vi "Main_MaintenanceCounters_EventDriven.vi"() -> ()   [LabVIEW 2017]
uses:
  <vilib>/Utility/file.llb/Write Delimited Spreadsheet (string).vi
panel:
  in  "SignaiFromPLC":bool[](array[boolean])
  out "CycleTimeCluster":T1
  out "Table Control":string[][](table)
  out "ConnectionCluster":cluster{"Connection":bool, "MachineName":string}
  out "UDT_1":T2
  in  "CountersConfiguration":T3
  out "CountersConfigMerged":T4(array[cluster])
  out "CounterLineName Path":path
  in  "stop":bool
  in  "Tab":T5(tab)
  in  "Sort":bool
  in  "ResetAlarm":bool[](array[boolean])
  out "ArrayAlarm":bool[](array[boolean])
  out "OnlineStations":T6(array[cluster])
  in  "Counters Monitor Array":T7(array[cluster])
  in  "RefreshCurrentCounter":bool
  in  "SaveCurrentCounter":bool
  out "CurrentCountersPath":path
  in  "Count Signal":bool[](array[boolean])
  out "CycleTimeMonitor":T8(array[cluster])
  out "CycleTimePath":path
  in  "CountersConfigArray":T4(array[cluster]) {"StoppageAlarmCounter" format="%#_6f"; "PreparationAlarmCounter" format="%#_6f"}
  in  "RefreshCountersConfig":bool
  in  "SaveCountersConfig":bool
  out "Counters Configuration Path":path
  in  "MachineNameID":u16(ring) items=["MA520", "MA500", "MA490", "MA475", "MA470"]
  out "Red":dbl
  out "Yellow":dbl
  out "Green":dbl
  out "Line Name":string
  in  "PLC Connection Array":T9(array[cluster]) {"MemoryType" items=["CR (Control Relay)", "MR (Internal Auxiliary Relay)", "VB (Work Relay)", "LR (Latch Relay)", "B (Link Relay)", "R (Relay)", "DM (Data Memory)", "EM (Extended Data Memory)", "FM (File Register 1)", "ZF (FIle Register 2)", "W (Link Register)", "TM (Temporary Data Memory)", "Z (Index Register)", "T (Timer)", "TC (Timer (Counter Value))", "TS (Timer Set Value)", "C (Counter)", "CC (Counter (Counter Value))", "CS (Counter (Set Value))", "CTH (High Speed Counter)", "CTC (High Speed Counter Comparator (Set Value))", "AT (Digital Trimmer)", "CM (Control Memory)", "VM (Work Memory)"]; "PLC Type" items=["Keyence", "Allen Bradley", "Mitsubishi", "Panasonic", "Siemens"]}
  in  "SavePLCConfig":bool
  in  "RefreshPLCConfig":bool
  out "PLC Configuration Path":path
  in  "EmailsEnabled":bool
  in  "MailConfigPath":path
  in  "MailConfigCluster":T10
  in  "AccessLevel":string
  in  "Role":string
  in  "Password":string
  in  "User":string
  in  "RefreshMailConfig":bool
  in  "SaveMailConfig":bool
  # "Cycles Based Maintenance"
  # "1. Save counters to be loaded in the last state when the app starts up.\n\n2.Algorithm to read PLC counter values.\nthe key will be to set the signal from the PLC and reset from LabVIEW and the machine won't be able to start the new signal if the application has not been reset the previous one.\n\n3. Autosort getting the red status all the way up.\n\n4. Check cyle time between parts (The count signal must is the same for all the components in the same machine)"
  # "Under Construction"
  # "Online Stations"
  # "MachineName"
  # "Tool Crib"
  # "ComponentName"
  # "SP1"
  # "Actual"
  # "Cycle Time Monitor"
  # "ToolCrib Part Number"
  # "MachineName"
  # "ComponentName"
  # "SP1"
  # "SP2"
  # "Note: \nTo add a machine in this list it must be firt added in the PLC\nConnection tab."
  # "Note:\nSP1 = Is the setpoint for the counter when the \nmachine will alert to prepare the replacement of\nthe component. This gives the technician time\nto get parts together.\n\nSP2 = Is the setpoint for the counter when the\nmachine will stop the operation until the part is \nreplaced, the operation can only be reset until\na quality employee comes to unlock with its \nuser and password."
  # "MachineName"
  # "PLC Address"
  # "PLC Type"
  # "Memory Type"
  # "MemoryNumber"
  # "Note:\nFor the PLC Connection I don't need a single bit, but a whole structure like the TM. \n\nStructure Example:\nEnd Cycle - Count Bit - Bool\nAlarm Bit - Stoppage Signal - Bool\nMessage - This is going to be a string that will transmit a message like 'Machine Stopped to Replace Electrodes'\n\nThe program will need to record in a log the time it stopped and the time the machine started production."
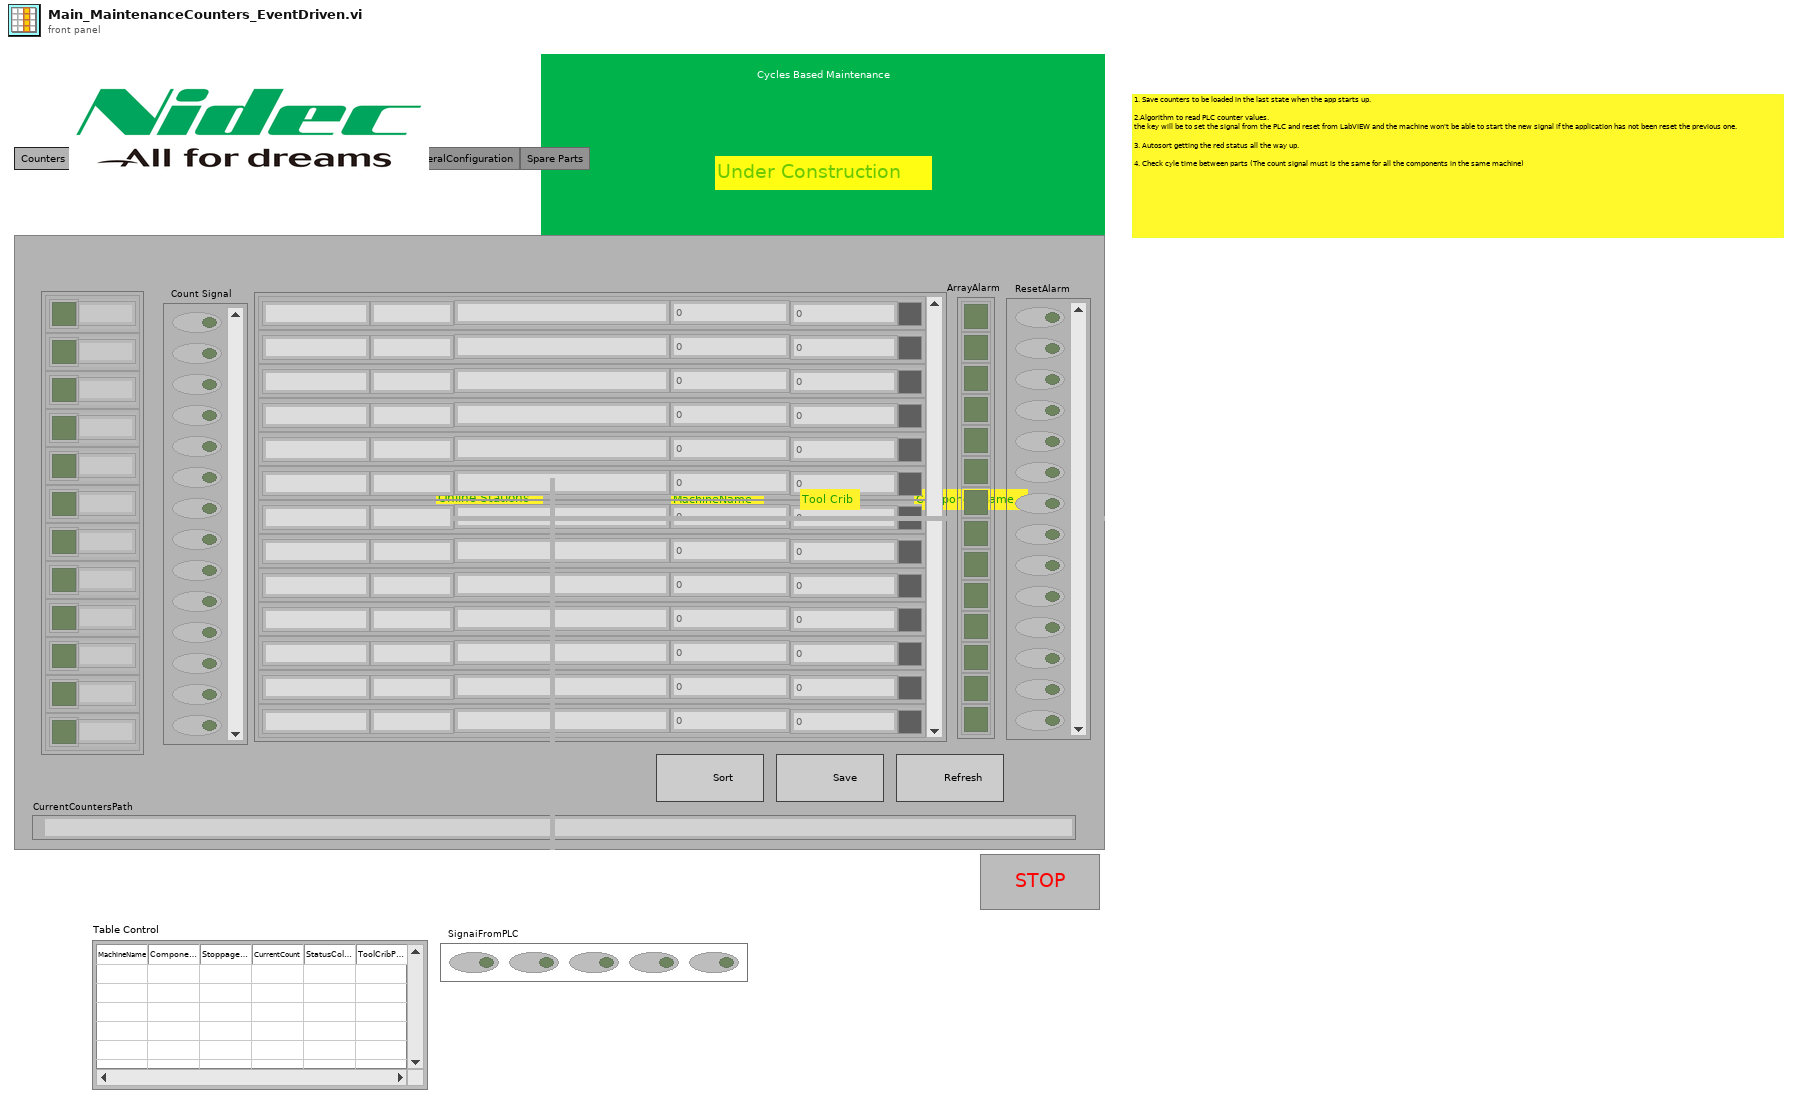
[diagram p1: front panel]
types:
  T1 = cluster{"Connection":bool, "MachineName":string, "CycleTime":dbl}
  T2 = cluster{"ToolCribPartNumber":string, "ComponentName":string, "PreparationAlarmCounter":dbl, "StoppageAlarmCounter":dbl, "MachineName":string}
  T3 = cluster{"MachineName":string, "ComponentName":string, "StoppageAlarmCounter":dbl, "CurrentCount":dbl, "StatusColorBox":u32, "ToolCribPartNumber":string}
  T4 = cluster{"ToolCribPartNumber":string, "ComponentName":string, "PreparationAlarmCounter":dbl, "StoppageAlarmCounter":dbl}[]
  T5 = enum32{"Counters Monitor", "CycleTime", "Counters Configuration", "PLC Connection", "GeneralConfiguration", "Spare Parts"}
  T6 = cluster{"Connection":bool, "MachineName":string}[]
  T7 = cluster{"MachineName":string, "ComponentName":string, "StoppageAlarmCounter":i32, "CurrentCount":i32, "StatusColorBox":u32, "ToolCribPartNumber":string}[]
  T8 = cluster{"Connection":bool, "MachineName":string, "CycleTime":dbl}[]
  T9 = cluster{"MachineName":string, "PLC Address":string, "PLC Type":u16, "MemoryType":u16, "MemoryNumber":i32}[]
  T10 = cluster{"MailSender":string, "MailPassword":string, "MailRecipients":string}
  T11 = cluster{"ToolCribPartNumber":string, "ComponentName":string, "PreparationAlarmCounter":dbl, "StoppageAlarmCounter":dbl, "MachineName":string}[]
  T12 = cluster{"MachineName":string, "ComponentName":string, "StoppageAlarmCounter":i32, "CurrentCount":i32, "StatusColorBox":u32, "ToolCribPartNumber":string}
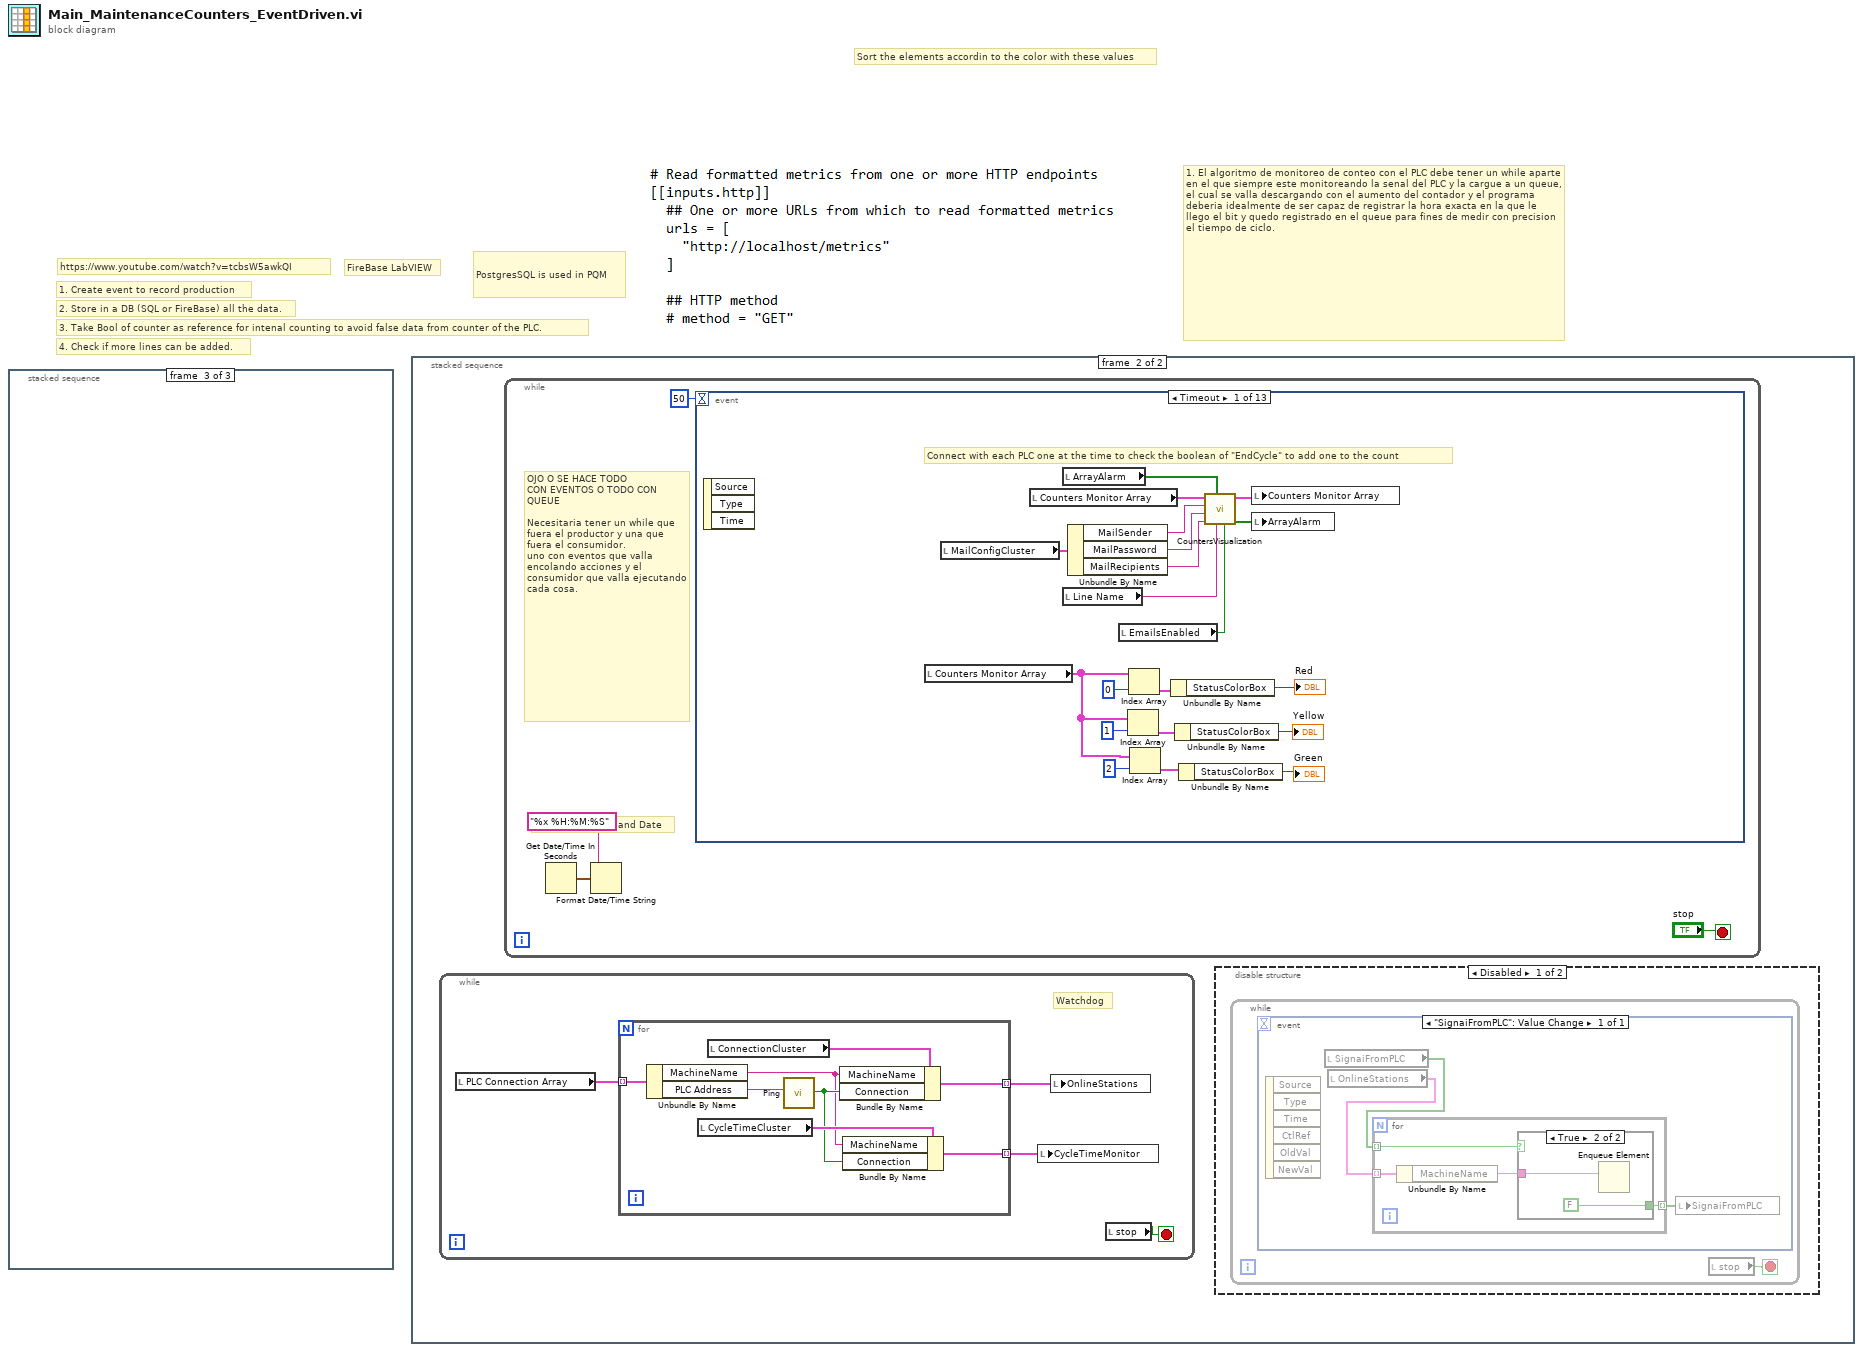
[diagram p0: block diagram]
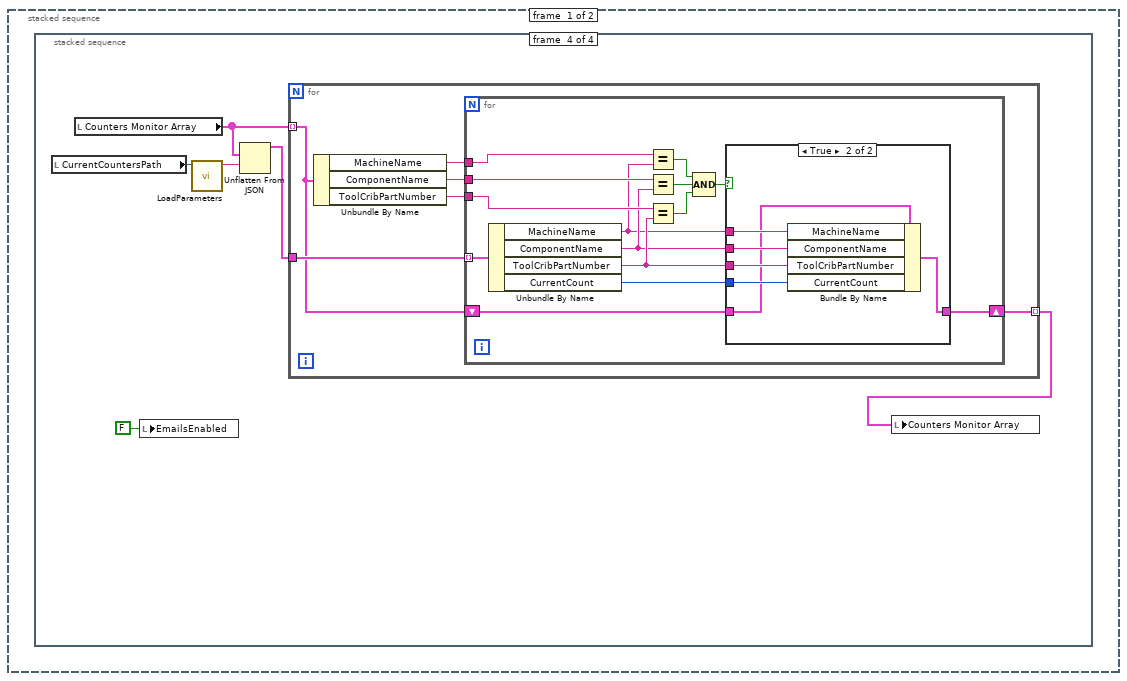
[diagram p2: hidden frame]
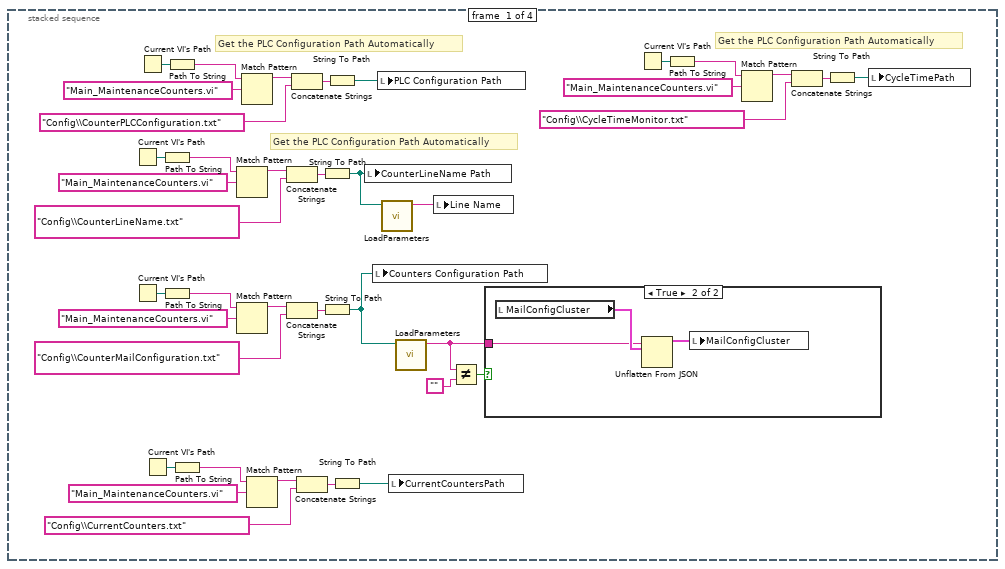
[diagram p3: hidden frame]
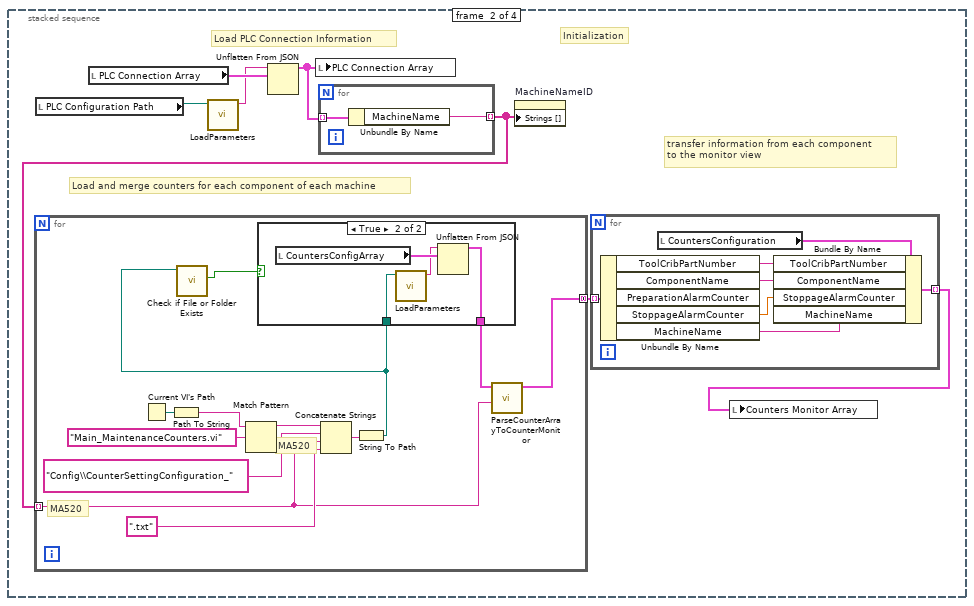
[diagram p5: hidden frame]
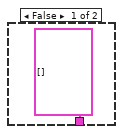
[diagram p6: hidden frame]
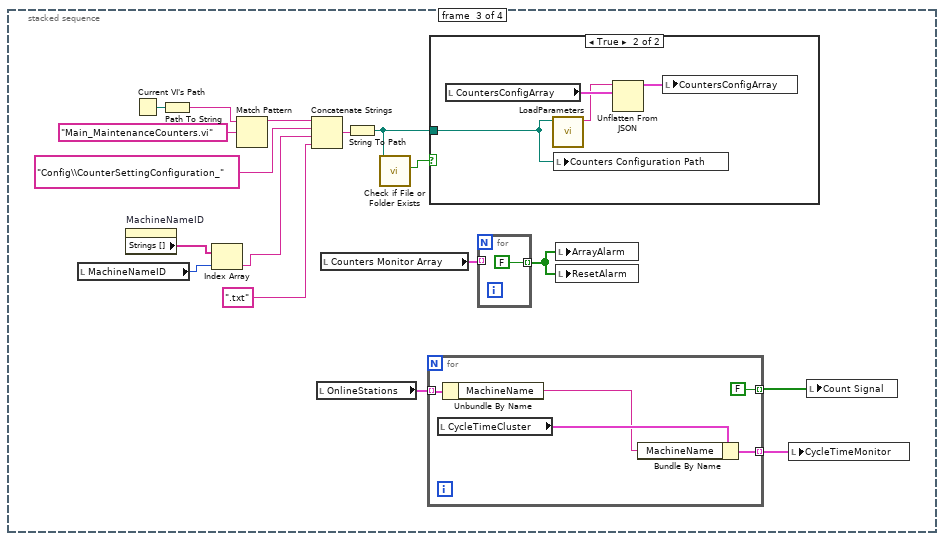
[diagram p7: hidden frame]
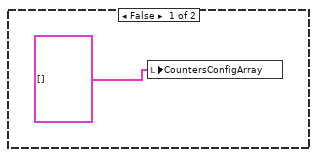
[diagram p8: hidden frame]
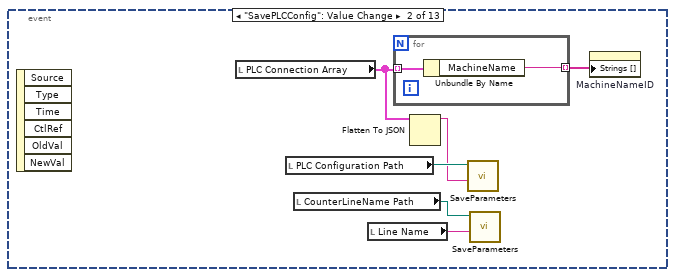
[diagram p12: hidden frame]
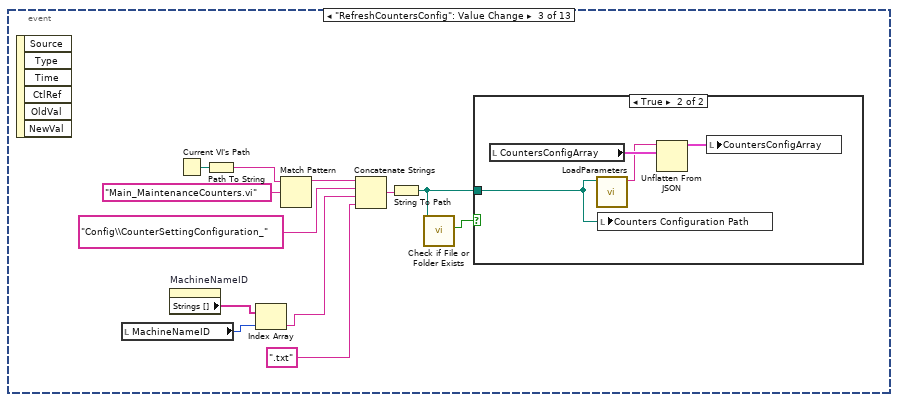
[diagram p13: hidden frame]
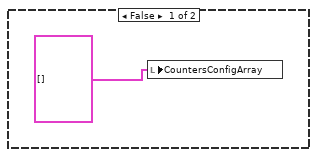
[diagram p14: hidden frame]
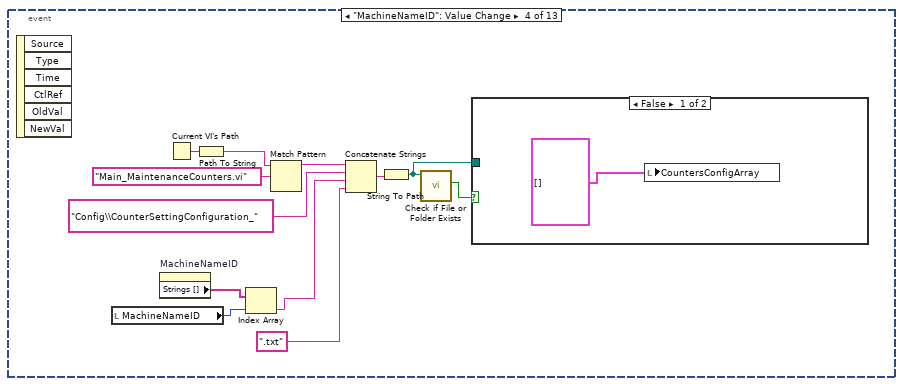
[diagram p15: hidden frame]
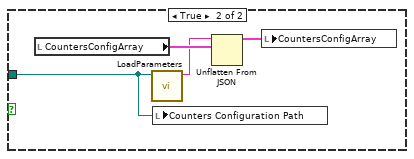
[diagram p16: hidden frame]
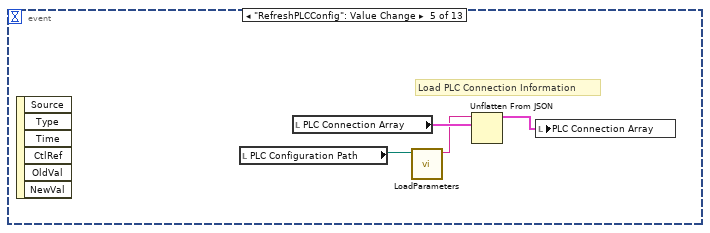
[diagram p17: hidden frame]
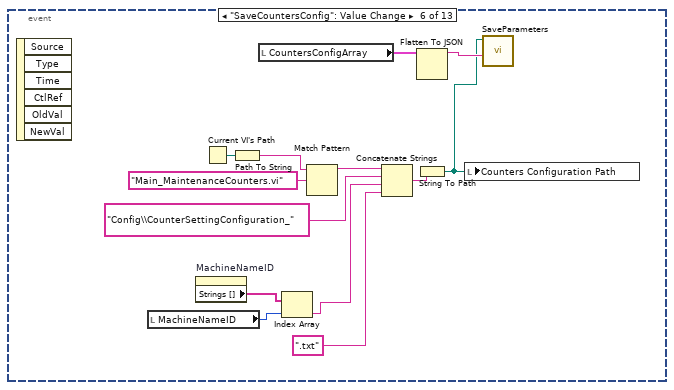
[diagram p18: hidden frame]
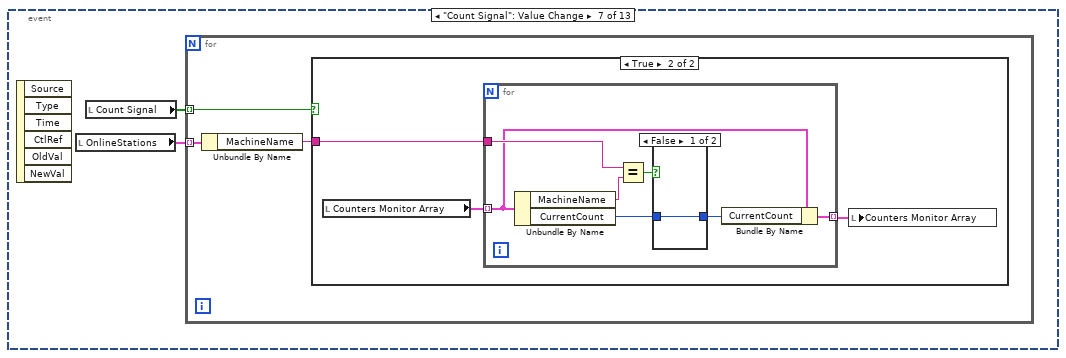
[diagram p19: hidden frame]
diagram:
  # "PostgresSQL is used in PQM"
  # "1. El algoritmo de monitoreo de conteo con el PLC debe tener un while aparte en el que siempre este monitoreando la senal del PLC y la cargue a un queue, el cual se valla descargando con el aumento del contador y el programa deberia idealmente de ser capaz de registrar la hora exacta en la que le llego el bit y quedo registrado en el queue para fines de medir con precision el tiempo de ciclo."
  # "Sort the elements accordin to the color with these values"
  # "FireBase LabVIEW"
  # "https://www.youtube.com/watch?v=tcbsW5awkQI"
  # "4. Check if more lines can be added."
  # "2. Store in a DB (SQL or FireBase) all the data."
  # "1. Create event to record production"
  # "3. Take Bool of counter as reference for intenal counting to avoid false data from counter of the PLC."
  n1 = stacked-sequence {
    frame #0 {
      w4 = FALSE
      # "Main Board"
      n2 = property on="CountersConfiguration" class="Clust (strict)"("Visible"=w4) -> ()  [unwired: 2 in, 2 out]
      n3 = property on="CountersConfigMerged" class="Arr (strict)"("Visible"=w4) -> ()  [unwired: 2 in, 2 out]
      n4 = property on="CounterLineName Path" class="Path"("Visible"=FALSE) -> ()  [unwired: 2 in, 2 out]
      n5 = property on="ConnectionCluster" class="Clust (strict)"("Visible"=FALSE) -> ()  [unwired: 2 in, 2 out]
      n6 = local write "stop"(FALSE ("stop")) -> ()
      n7 = property on="UDT_1" class="Clust (strict)"("Visible"=FALSE) -> ()  [unwired: 2 in, 2 out]
    }
    frame #1 {
      # "Configuration"
      n8 = property on="CycleTimeCluster" class="Clust (strict)"("Visible"=FALSE) -> ()  [unwired: 2 in, 2 out]
    }
    frame #2 {
    }
  }
  n9 = stacked-sequence {
    frame #0 {
      n10 = stacked-sequence {
        frame #0 {
          # "Get the PLC Configuration Path Automatically"
          # "Get the PLC Configuration Path Automatically"
          # "Get the PLC Configuration Path Automatically"
          n11 = Current VI's Path() -> (path=w38:path)
          n12 = Current VI's Path() -> (path=w25:path)
          n13 = Current VI's Path() -> (path=w45:path)
          n14 = Current VI's Path() -> (path=w14:path)
          n15 = Path To String(path=w38) -> (string=w37:string)
          n16 = Path To String(path=w25) -> (string=w26:string)
          n17 = Path To String(path=w45) -> (string=w44:string)
          n18 = Path To String(path=w14) -> (string=w15:string)
          n19 = Match Pattern(string=w37, regular expression="Main_MaintenanceCounters.vi") -> (before substring=w36:string)  [unwired: 1 in, 3 out]
          n20 = Match Pattern(string=w26, regular expression="Main_MaintenanceCounters.vi") -> (before substring=w27:string)  [unwired: 1 in, 3 out]
          n21 = Match Pattern(string=w44, regular expression="Main_MaintenanceCounters.vi") -> (before substring=w43:string)  [unwired: 1 in, 3 out]
          n22 = Match Pattern(string=w15, regular expression="Main_MaintenanceCounters.vi") -> (before substring=w16:string)  [unwired: 1 in, 3 out]
          n23 = Concatenate Strings(w36, "Config\\CounterLineName.txt" ("regular expression")) -> (w35:string)
          n24 = Concatenate Strings(w27, "Config\\CounterMailConfiguration.txt" ("regular expression")) -> (w28:string)
          n25 = Concatenate Strings(w43, "Config\\CounterPLCConfiguration.txt" ("regular expression")) -> (w42:string)
          n26 = Concatenate Strings(w16, "Config\\CurrentCounters.txt" ("regular expression")) -> (w17:string)
          n27 = String To Path(string=w35) -> (path=w32:path)
          n28 = String To Path(string=w28) -> (path=w24:path)
          n29 = String To Path(string=w42) -> (path=w41:path)
          n30 = String To Path(string=w17) -> (path=w18:path)
          n31 = local write "CounterLineName Path"(w32) -> ()
          n32 = local write "Counters Configuration Path"(w24) -> ()
          n33 = local write "PLC Configuration Path"(w41) -> ()
          n34 = call "LoadParameters.vi"("ShiftConfigPath"=w32) -> ("JSON_Text"=w31:string)  [unwired: 10 in]
          n35 = local write "CurrentCountersPath"(w18) -> ()
          n36 = call "LoadParameters.vi"("ShiftConfigPath"=w24) -> ("JSON_Text"=w23:string)  [unwired: 10 in]
          n37 = local write "Line Name"(w31) -> ()
          n38 = Not Equal?(x=w23, y="") -> (x != y?=w21:bool)
          n39 = case shown="True" w21 {
            tunnel: w23 -> [_ w46]
            frame False {
            }
            frame True {
              n40 = local read "MailConfigCluster"() -> (w48:T10)
              n41 = Unflatten From JSON(JSON string=w46, type and defaults=w48) -> (value=w47:T10)  [unwired: 5 in, 1 out]
              n42 = local write "MailConfigCluster"(w47) -> ()
            }
          }
          n43 = Current VI's Path() -> (path=w8:path)
          n44 = Path To String(path=w8) -> (string=w9:string)
          n45 = Match Pattern(string=w9, regular expression="Main_MaintenanceCounters.vi") -> (before substring=w10:string)  [unwired: 1 in, 3 out]
          n46 = Concatenate Strings(w10, "Config\\CycleTimeMonitor.txt" ("regular expression")) -> (w11:string)
          n47 = String To Path(string=w11) -> (path=w12:path)
          n48 = local write "CycleTimePath"(w12) -> ()
        }
        frame #1 {
          # "Initialization"
          # "transfer information from each component\nto the monitor view"
          # "Load and merge counters for each component of each machine"
          # "Load PLC Connection Information"
          n49 = local read "PLC Configuration Path"() -> (w54:path)
          n50 = local read "PLC Connection Array"() -> (w55:T9)
          n51 = call "LoadParameters.vi"("ShiftConfigPath"=w54) -> ("JSON_Text"=w53:string)  [unwired: 10 in]
          n52 = Unflatten From JSON(JSON string=w53, type and defaults=w55) -> (value=w52:T9)  [unwired: 5 in, 1 out]
          n53 = local write "PLC Connection Array"(w52) -> ()
          n54 = for {
            tunnel: w52 -> [w80] mode=indexing
            tunnel: [w81] -> w51 mode=indexing
            n55 = Unbundle By Name(w80) -> ("MachineName"=w81:string)
          }
          n56 = for {
            tunnel: w51 -> [w66] mode=indexing
            tunnel: [w65] -> w49 mode=concatenating
            # "MA520"
            # "MA520"
            n57 = Current VI's Path() -> (path=w71:path)
            n58 = Path To String(path=w71) -> (string=w72:string)
            n59 = Match Pattern(string=w72, regular expression="Main_MaintenanceCounters.vi") -> (before substring=w73:string)  [unwired: 1 in, 3 out]
            n60 = Concatenate Strings(w73, "Config\\CounterSettingConfiguration_" ("regular expression"), w66, ".txt" ("regular expression")) -> (w74:string)
            n61 = String To Path(string=w74) -> (path=w64:path)
            n62 = call <vilib>:"Check if File or Folder Exists.vi"("path"=w64) -> ("file or folder exists?"=w63:bool)  [unwired: 8 in, 2 out]
            n63 = case shown="True" w63 {
              tunnel: [T4 [] ("CountersConfigArray") w77] -> w67
              tunnel: w64 -> [_ w76]
              frame False {
              }
              frame True {
                n64 = local read "CountersConfigArray"() -> (w79:T4)
                n65 = call "LoadParameters.vi"("ShiftConfigPath"=w76) -> ("JSON_Text"=w78:string)  [unwired: 10 in]
                n66 = Unflatten From JSON(JSON string=w78, type and defaults=w79) -> (value=w77:T4)  [unwired: 5 in, 1 out]
              }
            }
            n67 = call "ParseCounterArrayToCounterMonitor.vi"("MachineID"=w66, "CountersConfigArray"=w67) -> ("CounterMonitorArray"=w65:T11)  [unwired: 9 in]
          }
          n68 = property on="MachineNameID" class="Ring (strict)"("Strings []"=w51) -> ()  [unwired: 2 in, 2 out]
          n69 = for {
            tunnel: [w60] -> w50 mode=indexing
            tunnel: w49 -> [w59] mode=indexing
            n70 = Unbundle By Name(w59) -> ("ToolCribPartNumber"=w58:string, "ComponentName"=w61:string, "StoppageAlarmCounter"=w57:dbl, "MachineName"=w56:string)  [unwired: 1 out]
            n71 = local read "CountersConfiguration"() -> (w62:T3)
            n72 = Bundle By Name(cluster=w62, "ToolCribPartNumber"=w58, "ComponentName"=w61, "StoppageAlarmCounter"=w57, "MachineName"=w56) -> (w60:T3)
          }
          n73 = local write "Counters Monitor Array"(w50) -> ()
        }
        frame #2 {
          n74 = local read "MachineNameID"() -> (w98:u16)
          n75 = property on="MachineNameID" class="Ring (strict)"() -> ("Strings []"=w97:string[])  [unwired: 2 in, 2 out]
          n76 = Current VI's Path() -> (path=w93:path)
          n77 = Path To String(path=w93) -> (string=w94:string)
          n78 = Index Array(array=w97, index=w98) -> (element=w92:string)
          n79 = Match Pattern(string=w94, regular expression="Main_MaintenanceCounters.vi") -> (before substring=w95:string)  [unwired: 1 in, 3 out]
          n80 = Concatenate Strings(w95, "Config\\CounterSettingConfiguration_" ("regular expression"), w92, ".txt" ("regular expression")) -> (w96:string)
          n81 = local read "OnlineStations"() -> (w84:T6)
          n82 = local read "Counters Monitor Array"() -> (w86:T7)
          n83 = String To Path(string=w96) -> (path=w90:path)
          n84 = call <vilib>:"Check if File or Folder Exists.vi"("path"=w90) -> ("file or folder exists?"=w91:bool)  [unwired: 8 in, 2 out]
          n85 = for {
            tunnel: w84 -> [w101] mode=indexing
            tunnel: [FALSE] -> w83 mode=indexing
            tunnel: [w99] -> w82 mode=indexing
            n86 = local read "CycleTimeCluster"() -> (w102:T1)
            n87 = Unbundle By Name(w101) -> ("MachineName"=w100:string)
            n88 = Bundle By Name(cluster=w102, "MachineName"=w100) -> (w99:T1)
          }
          n89 = case shown="True" w91 {
            tunnel: w90 -> [_ w106]
            frame False {
              n90 = local write "CountersConfigArray"(T4 [] ("CountersConfigArray")) -> ()
            }
            frame True {
              n91 = local read "CountersConfigArray"() -> (w109:T4)
              n92 = call "LoadParameters.vi"("ShiftConfigPath"=w106) -> ("JSON_Text"=w107:string)  [unwired: 10 in]
              n93 = local write "Counters Configuration Path"(w106) -> ()
              n94 = Unflatten From JSON(JSON string=w107, type and defaults=w109) -> (value=w108:T4)  [unwired: 5 in, 1 out]
              n95 = local write "CountersConfigArray"(w108) -> ()
            }
          }
          n96 = for {
            tunnel: w86 -> [_] mode=indexing
            tunnel: [FALSE] -> w85 mode=indexing
          }
          n97 = local write "ArrayAlarm"(w85) -> ()
          n98 = local write "ResetAlarm"(w85) -> ()
          n99 = local write "CycleTimeMonitor"(w82) -> ()
          n100 = local write "Count Signal"(w83) -> ()
        }
        frame #3 {
          n101 = local read "CurrentCountersPath"() -> (w115:path)
          n102 = local read "Counters Monitor Array"() -> (w113:T7)
          n103 = local write "EmailsEnabled"(FALSE ("EmailsEnabled")) -> ()
          n104 = call "LoadParameters.vi"("ShiftConfigPath"=w115) -> ("JSON_Text"=w114:string)  [unwired: 10 in]
          n105 = Unflatten From JSON(JSON string=w114, type and defaults=w113) -> (value=w112:T7)  [unwired: 5 in, 1 out]
          n106 = for {
            tunnel: w113 -> [w117] mode=indexing
            tunnel: w112 -> [w118]
            tunnel: [w116] -> w111 mode=indexing
            n107 = Unbundle By Name(w117) -> ("MachineName"=w121:string, "ComponentName"=w120:string, "ToolCribPartNumber"=w119:string)
            n108 = for {
              tunnel: w121 -> [w134]
              tunnel: w120 -> [w133]
              tunnel: w119 -> [w132]
              tunnel: w118 -> [w135] mode=indexing
              shift-right: [w122] -> w116
              shift-left: w117 -> [w123]
              n109 = Unbundle By Name(w135) -> ("MachineName"=w124:string, "ComponentName"=w125:string, "ToolCribPartNumber"=w126:string, "CurrentCount"=w128:i32)
              n110 = Equal?(x=w134, y=w124) -> (x = y?=w130:bool)
              n111 = Equal?(x=w133, y=w125) -> (x = y?=w131:bool)
              n112 = Equal?(x=w132, y=w126) -> (x = y?=w129:bool)
              n113 = Compound Arithmetic op=AND(w130, w131, w129) -> (w127:bool)
              n114 = case shown="True" w127 {
                tunnel: w128 -> [_ w142]
                tunnel: w126 -> [_ w141]
                tunnel: w125 -> [_ w140]
                tunnel: w124 -> [_ w139]
                tunnel: w123 -> [w136 w138]
                tunnel: [w136 w137] -> w122
                frame False {
                }
                frame True {
                  n115 = Bundle By Name(cluster=w138, "MachineName"=w139, "ComponentName"=w140, "ToolCribPartNumber"=w141, "CurrentCount"=w142) -> (w137:T12)
                }
              }
            }
          }
          n116 = local write "Counters Monitor Array"(w111) -> ()
        }
      }
    }
    frame #1 {
      n117 = while {
        stop <- w146 stop-if-true
        # "Watchdog"
        n118 = local read "PLC Connection Array"() -> (w144:T9)
        n119 = for {
          tunnel: w144 -> [w154] mode=indexing
          tunnel: [w151] -> w145 mode=indexing
          tunnel: [w147] -> w143 mode=indexing
          n120 = Unbundle By Name(w154) -> ("MachineName"=w148:string, "PLC Address"=w153:string)
          n121 = local read "CycleTimeCluster"() -> (w150:T1)
          n122 = local read "ConnectionCluster"() -> (w152:cluster{"Connection":bool, "MachineName":string})
          n123 = call "Ping.vi"("hostNameOrAddress"=w153) -> ("bolStatus"=w149:bool)  [unwired: 8 in, 2 out]
          n124 = Bundle By Name(cluster=w152, "MachineName"=w148, "Connection"=w149) -> (w151:cluster{"Connection":bool, "MachineName":string})
          n125 = Bundle By Name(cluster=w150, "MachineName"=w148, "Connection"=w149) -> (w147:T1)
        }
        n126 = local write "CycleTimeMonitor"(w143) -> ()
        n127 = local write "OnlineStations"(w145) -> ()
        n128 = local read "stop"() -> (w146:bool)
      }
      n129 = while {
        stop <- "stop" stop-if-true
        # "OJO O SE HACE TODO\nCON EVENTOS O TODO CON\nQUEUE \n\nNecesitaria tener un while que fuera el productor y una que fuera el consumidor.\nuno con eventos que valla encolando acciones y el consumidor que valla ejecutando cada cosa."
        # "Get current Hour and Date"
        n130 = Get Date/Time In Seconds() -> (seconds since 1Jan1904=w168:timestamp)
        n131 = Format Date/Time String(time format string (%c)="%x %H:%M:%S", seconds (now)=w168) -> ()  [unwired: 1 in, 1 out]
        n132 = event shown="[0] Timeout" {
          selector: _ -> [_ _ _ _ _ _ _ _ _ _ _ _ _]
          dyn-events: _ -> [_ _ _ _ _ _ _ _ _ _ _ _ _]
          timeout: 50 -> [_ _ _ _ _ _ _ _ _ _ _ _ _]
          event Timeout {
            # "Connect with each PLC one at the time to check the boolean of \"EndCycle\" to add one to the count"
            n133 = event-data() -> ()  [unwired: 1 in, 3 out]
            n134 = local read "Counters Monitor Array"() -> (w170:T7)
            n135 = local read "MailConfigCluster"() -> (w186:T10)
            n136 = local read "Counters Monitor Array"() -> (w189:T7)
            n137 = local read "ArrayAlarm"() -> (w182:bool[])
            n138 = local read "Line Name"() -> (w187:string)
            n139 = Unbundle By Name(w186) -> ("MailSender"=w185:string, "MailPassword"=w184:string, "MailRecipients"=w183:string)
            n140 = local read "EmailsEnabled"() -> (w171:bool)
            n141 = Index Array(array=w170, index=1) -> (element=w175:T12)
            n142 = Index Array(array=w170, index=0) -> (element=w177:T12)
            n143 = Index Array(array=w170, index=2) -> (element=w176:T12)
            n144 = Unbundle By Name(w177) -> ("StatusColorBox"=→"Red":u32)
            n145 = Unbundle By Name(w175) -> ("StatusColorBox"=→"Yellow":u32)
            n146 = Unbundle By Name(w176) -> ("StatusColorBox"=→"Green":u32)
            n147 = call "CountersVisualization.vi"("EmailEnabled"=w171, "LineName"=w187, "ArrayAlarmIN"=w182, "Recipients"=w183, "Password"=w184, "SenderMail"=w185, "Counters Monitor Array IN"=w189) -> ("ArrayAlarmOUT"=w181:bool[], "Counters Monitor Array OUT"=w188:T7)  [unwired: 3 in]
            n148 = local write "Counters Monitor Array"(w188) -> ()
            n149 = local write "ArrayAlarm"(w181) -> ()
          }
          event "SavePLCConfig": Value Change {
            n150 = event-data() -> ()  [unwired: 1 in, 6 out]
            n151 = local read "PLC Connection Array"() -> (w194:T9)
            n152 = local read "PLC Configuration Path"() -> (w193:path)
            n153 = local read "CounterLineName Path"() -> (w190:path)
            n154 = local read "Line Name"() -> (w191:string)
            n155 = for {
              tunnel: w194 -> [w197] mode=indexing
              tunnel: [w196] -> w195 mode=indexing
              n156 = Unbundle By Name(w197) -> ("MachineName"=w196:string)
            }
            n157 = Flatten To JSON(anything=w194) -> (JSON string=w192:string)  [unwired: 2 in, 1 out]
            n158 = call "SaveParameters.vi"("JSON_Text"=w192, "ShiftConfigPath"=w193) -> ()  [unwired: 10 in]
            n159 = call "SaveParameters.vi"("JSON_Text"=w191, "ShiftConfigPath"=w190) -> ()  [unwired: 10 in]
            n160 = property on="MachineNameID" class="Ring (strict)"("Strings []"=w195) -> ()  [unwired: 2 in, 2 out]
          }
          event "RefreshCountersConfig": Value Change {
            n161 = event-data() -> ()  [unwired: 1 in, 6 out]
            n162 = local read "MachineNameID"() -> (w209:u16)
            n163 = property on="MachineNameID" class="Ring (strict)"() -> ("Strings []"=w208:string[])  [unwired: 2 in, 2 out]
            n164 = Current VI's Path() -> (path=w204:path)
            n165 = Path To String(path=w204) -> (string=w205:string)
            n166 = Index Array(array=w208, index=w209) -> (element=w203:string)
            n167 = Match Pattern(string=w205, regular expression="Main_MaintenanceCounters.vi") -> (before substring=w206:string)  [unwired: 1 in, 3 out]
            n168 = Concatenate Strings(w206, "Config\\CounterSettingConfiguration_" ("regular expression"), w203, ".txt" ("regular expression")) -> (w207:string)
            n169 = String To Path(string=w207) -> (path=w198:path)
            n170 = call <vilib>:"Check if File or Folder Exists.vi"("path"=w198) -> ("file or folder exists?"=w199:bool)  [unwired: 8 in, 2 out]
            n171 = case shown="True" w199 {
              tunnel: w198 -> [_ w211]
              frame False {
                n172 = local write "CountersConfigArray"(T4 [] ("CountersConfigArray")) -> ()
              }
              frame True {
                n173 = local read "CountersConfigArray"() -> (w214:T4)
                n174 = call "LoadParameters.vi"("ShiftConfigPath"=w211) -> ("JSON_Text"=w212:string)  [unwired: 10 in]
                n175 = local write "Counters Configuration Path"(w211) -> ()
                n176 = Unflatten From JSON(JSON string=w212, type and defaults=w214) -> (value=w213:T4)  [unwired: 5 in, 1 out]
                n177 = local write "CountersConfigArray"(w213) -> ()
              }
            }
          }
          event "MachineNameID": Value Change {
            n178 = event-data() -> ()  [unwired: 1 in, 6 out]
            n179 = local read "MachineNameID"() -> (w226:u16)
            n180 = property on="MachineNameID" class="Ring (strict)"() -> ("Strings []"=w225:string[])  [unwired: 2 in, 2 out]
            n181 = Current VI's Path() -> (path=w221:path)
            n182 = Path To String(path=w221) -> (string=w222:string)
            n183 = Index Array(array=w225, index=w226) -> (element=w220:string)
            n184 = Match Pattern(string=w222, regular expression="Main_MaintenanceCounters.vi") -> (before substring=w223:string)  [unwired: 1 in, 3 out]
            n185 = Concatenate Strings(w223, "Config\\CounterSettingConfiguration_" ("regular expression"), w220, ".txt" ("regular expression")) -> (w224:string)
            n186 = String To Path(string=w224) -> (path=w215:path)
            n187 = call <vilib>:"Check if File or Folder Exists.vi"("path"=w215) -> ("file or folder exists?"=w216:bool)  [unwired: 8 in, 2 out]
            n188 = case shown="False" w216 {
              tunnel: w215 -> [_ w228]
              frame False {
                n189 = local write "CountersConfigArray"(T4 [] ("CountersConfigArray")) -> ()
              }
              frame True {
                n190 = local read "CountersConfigArray"() -> (w231:T4)
                n191 = call "LoadParameters.vi"("ShiftConfigPath"=w228) -> ("JSON_Text"=w229:string)  [unwired: 10 in]
                n192 = local write "Counters Configuration Path"(w228) -> ()
                n193 = Unflatten From JSON(JSON string=w229, type and defaults=w231) -> (value=w230:T4)  [unwired: 5 in, 1 out]
                n194 = local write "CountersConfigArray"(w230) -> ()
              }
            }
          }
          event "RefreshPLCConfig": Value Change {
            # "Load PLC Connection Information"
            n195 = event-data() -> ()  [unwired: 1 in, 6 out]
            n196 = local read "PLC Configuration Path"() -> (w233:path)
            n197 = local read "PLC Connection Array"() -> (w234:T9)
            n198 = call "LoadParameters.vi"("ShiftConfigPath"=w233) -> ("JSON_Text"=w232:string)  [unwired: 10 in]
            n199 = Unflatten From JSON(JSON string=w232, type and defaults=w234) -> (value=w235:T9)  [unwired: 5 in, 1 out]
            n200 = local write "PLC Connection Array"(w235) -> ()
          }
          event "SaveCountersConfig": Value Change {
            n201 = event-data() -> ()  [unwired: 1 in, 6 out]
            n202 = local read "MachineNameID"() -> (w248:u16)
            n203 = property on="MachineNameID" class="Ring (strict)"() -> ("Strings []"=w247:string[])  [unwired: 2 in, 2 out]
            n204 = Current VI's Path() -> (path=w243:path)
            n205 = Path To String(path=w243) -> (string=w244:string)
            n206 = local read "CountersConfigArray"() -> (w238:T4)
            n207 = Index Array(array=w247, index=w248) -> (element=w240:string)
            n208 = Match Pattern(string=w244, regular expression="Main_MaintenanceCounters.vi") -> (before substring=w245:string)  [unwired: 1 in, 3 out]
            n209 = Concatenate Strings(w245, "Config\\CounterSettingConfiguration_" ("regular expression"), w240, ".txt" ("regular expression")) -> (w246:string)
            n210 = Flatten To JSON(anything=w238) -> (JSON string=w237:string)  [unwired: 2 in, 1 out]
            n211 = String To Path(string=w246) -> (path=w236:path)
            n212 = local write "Counters Configuration Path"(w236) -> ()
            n213 = call "SaveParameters.vi"("JSON_Text"=w237, "ShiftConfigPath"=w236) -> ()  [unwired: 10 in]
          }
          event "Count Signal": Value Change {
            n214 = event-data() -> ()  [unwired: 1 in, 6 out]
            n215 = local read "OnlineStations"() -> (w249:T6)
            n216 = local read "Count Signal"() -> (w250:bool[])
            n217 = for {
              tunnel: w250 -> [w252] mode=indexing
              tunnel: w249 -> [w253] mode=indexing
              n218 = Unbundle By Name(w253) -> ("MachineName"=w251:string)
              n219 = case shown="True" w252 {
                tunnel: w251 -> [_ w255]
                frame False {
                }
                frame True {
                  n220 = local read "Counters Monitor Array"() -> (w256:T7)
                  n221 = for {
                    tunnel: w256 -> [w259] mode=indexing
                    tunnel: w255 -> [w262]
                    tunnel: [w257] -> w254 mode=indexing
                    n222 = Unbundle By Name(w259) -> ("MachineName"=w263:string, "CurrentCount"=w260:i32)
                    n223 = Equal?(x=w262, y=w263) -> (x = y?=w261:bool)
                    n224 = case shown="False" w261 {
                      tunnel: w260 -> [w264 w266]
                      tunnel: [w264 w265] -> w258
                      frame False {
                      }
                      frame True {
                        n225 = Increment(x=w266) -> (x+1=w265:i32)
                      }
                    }
                    n226 = Bundle By Name(cluster=w259, "CurrentCount"=w258) -> (w257:T12)
                  }
                  n227 = local write "Counters Monitor Array"(w254) -> ()
                }
              }
            }
          }
          event "ResetAlarm": Value Change {
            n228 = event-data() -> ()  [unwired: 1 in, 6 out]
            n229 = local read "Counters Monitor Array"() -> (w268:T7)
            n230 = local read "ResetAlarm"() -> (w271:bool[])
            n231 = local read "ArrayAlarm"() -> (w270:bool[])
            n232 = for {
              tunnel: w271 -> [w277] mode=indexing
              tunnel: w270 -> [w274] mode=indexing
              tunnel: [w275] -> w269 mode=indexing
              tunnel: w268 -> [w272] mode=indexing
              tunnel: [w273] -> w267 mode=indexing
              n233 = And(x=w277, y=w274) -> (x .and. y?=w276:bool)
              n234 = case shown="True" w276 {
                tunnel: [w279 FALSE] -> w275
                tunnel: w274 -> [w279 _]
                tunnel: w272 -> [w278 _]
                tunnel: [w278 w280] -> w273
                tunnel: w272 -> [_ w282]
                frame False {
                }
                frame True {
                  n235 = Bundle By Name(cluster=w282, "CurrentCount"=0) -> (w280:T12)
                }
              }
            }
            n236 = local write "ArrayAlarm"(w269) -> ()
            n237 = local write "Counters Monitor Array"(w267) -> ()
          }
          event "SaveMailConfig": Value Change {
            n238 = event-data() -> ()  [unwired: 1 in, 6 out]
            n239 = local read "MailConfigCluster"() -> (w285:T10)
            n240 = local read "MailConfigPath"() -> (w286:path)
            n241 = Flatten To JSON(anything=w285) -> (JSON string=w284:string)  [unwired: 2 in, 1 out]
            n242 = call "SaveParameters.vi"("JSON_Text"=w284, "ShiftConfigPath"=w286) -> ()  [unwired: 10 in]
          }
          event "RefreshMailConfig": Value Change {
            n243 = event-data() -> ()  [unwired: 1 in, 6 out]
            n244 = local read "Counters Configuration Path"() -> (w290:path)
            n245 = local read "MailConfigCluster"() -> (w288:T10)
            n246 = call "LoadParameters.vi"("ShiftConfigPath"=w290) -> ("JSON_Text"=w289:string)  [unwired: 10 in]
            n247 = Unflatten From JSON(JSON string=w289, type and defaults=w288) -> (value=w287:T10)  [unwired: 5 in, 1 out]
            n248 = local write "MailConfigCluster"(w287) -> ()
          }
          event "SaveCurrentCounter": Value Change {
            w291 = "," ("delimiter (\\t)")
            n249 = event-data() -> ()  [unwired: 1 in, 6 out]
            n250 = property on="Table Control" class="Tbl (strict)"() -> ("Column Headers[]"=w295:string[])  [unwired: 2 in, 2 out]
            n251 = local read "Counters Monitor Array"() -> (w298:T7)
            n252 = call-poly <vilib>:"Write Delimited Spreadsheet.vi"("file path (dialog if empty)"=path "C:/VSD/ProductionMonitor/InfluxDB_DirectoryMonitor/ReadFilesFromHere/CurrentCounters.csv", "1D data"=w295, "delimiter (\\t)"=w291) -> ("new file path (Not A Path if cancelled)"=w293:path, "error out"=w294:errorcluster)  [unwired: 11 in]
            n253 = local read "CurrentCountersPath"() -> (w300:path)
            n254 = local read "Table Control"() -> (w297:string[][])
            n255 = Flatten To JSON(anything=w298) -> (JSON string=w299:string)  [unwired: 2 in, 1 out]
            n256 = call-poly <vilib>:"Write Delimited Spreadsheet.vi"("file path (dialog if empty)"=w293, "2D data"=w297, "append to file? (new file:F)"=TRUE, "error in (no error)"=w294, "delimiter (\\t)"=w291) -> ()  [unwired: 9 in, 2 out]
            n257 = call "SaveParameters.vi"("JSON_Text"=w299, "ShiftConfigPath"=w300) -> ()  [unwired: 10 in]
          }
          event "RefreshCurrentCounter": Value Change {
            n258 = event-data() -> ()  [unwired: 1 in, 6 out]
            n259 = local read "CurrentCountersPath"() -> (w304:path)
            n260 = local read "Counters Monitor Array"() -> (w302:T7)
            n261 = call "LoadParameters.vi"("ShiftConfigPath"=w304) -> ("JSON_Text"=w303:string)  [unwired: 10 in]
            n262 = Unflatten From JSON(JSON string=w303, type and defaults=w302) -> (value=w301:T7)  [unwired: 5 in, 1 out]
            n263 = local write "Counters Monitor Array"(w301) -> ()
          }
          event "Sort": Value Change {
            n264 = event-data() -> ()  [unwired: 1 in, 6 out]
            n265 = local read "Counters Monitor Array"() -> (w314:T7)
            n266 = for {
              tunnel: w314 -> [w324] mode=indexing
              tunnel: [w323] -> w312 mode=indexing
              tunnel: [w322] -> w311 mode=indexing
              tunnel: [w320] -> w310 mode=indexing
              tunnel: [w318] -> w309 mode=indexing
              tunnel: [w316] -> w308 mode=indexing
              tunnel: [w315] -> w307 mode=indexing
              n267 = Unbundle By Name(w324) -> ("MachineName"=w323:string, "ComponentName"=w322:string, "StoppageAlarmCounter"=w321:i32, "CurrentCount"=w319:i32, "StatusColorBox"=w317:u32, "ToolCribPartNumber"=w315:string)
              n268 = Number To Decimal String(number=w321) -> (decimal integer string=w320:string)  [unwired: 1 in]
              n269 = Number To Decimal String(number=w319) -> (decimal integer string=w318:string)  [unwired: 1 in]
              n270 = Number To Decimal String(number=w317) -> (decimal integer string=w316:string)  [unwired: 1 in]
            }
            n271 = property on="Table Control" class="Tbl (strict)"("Column Headers[]"=string[] ["MachineName", "ComponentName", "StoppageCounter", "CurrentCount", "StatusColorBox", "ToolCribPartNumber"]) -> ()  [unwired: 2 in, 2 out]
            n272 = Build Array(w312, w311, w310, w309, w308, w307) -> (w306:string[][])
            n273 = Transpose 2D Array(2D array=w306) -> (transposed array=w305:string[][])
            n274 = local write "Table Control"(w305) -> ()
          }
        }
      }
      n275 = disable-structure shown="Disabled" {
        frame Disabled {
          n276 = while {
            stop <- w155 stop-if-true
            n277 = event shown="[0] \"SignaiFromPLC\": Value Change" {
              selector: _ -> [_]
              dyn-events: _ -> [_]
              timeout: _ -> [_]
              event "SignaiFromPLC": Value Change {
                n278 = event-data() -> ()  [unwired: 1 in, 6 out]
                n279 = local read "SignaiFromPLC"() -> (w157:bool[])
                n280 = local read "OnlineStations"() -> (w158:T6)
                n281 = for {
                  tunnel: w158 -> [w162] mode=indexing
                  tunnel: w157 -> [w160] mode=indexing
                  tunnel: [w159] -> w156 mode=indexing
                  n282 = Unbundle By Name(w162) -> ("MachineName"=w161:string)
                  n283 = case shown="True" w160 {
                    selector: w160 -> [w163 _]
                    tunnel: w161 -> [_ w165]
                    tunnel: [w163 FALSE] -> w159
                    frame False {
                    }
                    frame True {
                      n284 = Enqueue Element(element=w165) -> ()  [unwired: 3 in, 3 out]
                    }
                  }
                }
                n285 = local write "SignaiFromPLC"(w156) -> ()
              }
            }
            n286 = local read "stop"() -> (w155:bool)
          }
        }
        frame Enabled {
        }
      }
    }
  }
